vi "Fixed Point.vi"() -> (3 "Unit Test Framework Results":T1)   [LabVIEW 2015]
doc: "Use this template to create a user-defined test VI. Define your test requirements and wire the results to the <b>Result (Test)</b> control. Do not modify the <b>Unit Test Framework Results</b> indicator."
uses:
  <vilib>/utf/common/utf_test_result_troll.ctl
  <vilib>/utf/common/utf_test_result.ctl
  <vilib>/utf/common/utf_test_result_failure.ctl
  <vilib>/utf/common/utf_test_comparison_operators.ctl
  <vilib>/utf/common/utf_vi_tag.ctl
  <userlib>/LV Test Utils v1/LV Test Utils.lvlib
  <vilib>/utf/NI_UnitTestFramework.lvlib
panel:
  out "string":string
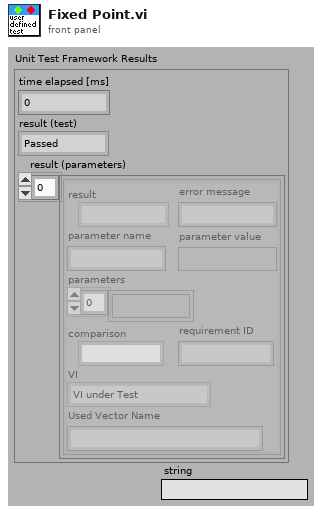
[diagram p1: front panel]
types:
  T1 = typedef "NI_UnitTestFramework.lvlib/utf_test_result_troll.ctl" = cluster{"time elapsed [ms]":u32, "result (test)":T2, "result (parameters)":T3[]}
  T2 = typedef "NI_UnitTestFramework.lvlib/utf_test_result.ctl" = enum16{"Passed", "Failed", "Error", "Skipped", "Not Processed"}
  T3 = typedef "NI_UnitTestFramework.lvlib/utf_test_result_failure.ctl" = cluster{"result":T2, "error message":string, "parameter name":string, "parameter value":variant, "parameters":variant[], "comparison":T4, "requirement ID":string, "VI":T5, "Used Vector Name":string}
  T4 = typedef "NI_UnitTestFramework.lvlib/utf_test_comparison_operators.ctl" = enum16{"=", "!=", ">", ">=", "<", "<=", "range", "symmetric tolerance", "asymmetric tolerance", "string contains", "string not contain", "array size", "string length", "array range", "by element", "array range (limit array)", "user-defined", "array contains", "array not contain", "vector length", "= (elm)", "!= (elm)", "= (case insensitive)", "!= (case insensitive)"}
  T5 = typedef "NI_UnitTestFramework.lvlib/utf_vi_tag.ctl" = enum16{"Setup VI", "VI under Test", "Teardown VI"}
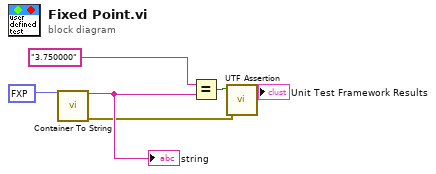
[diagram p0: block diagram]
diagram:
  n1 = call "Container To String.vi"("variant"=fxp<+,4,2> 3.75) -> ("string"=w5:string, "error out"=w2:errorcluster)  [unwired: 12 in, 1 out]
  "string" <- w5
  n2 = Equal?(x="3.750000" ("string"), y=w5) -> (x = y?=w3:bool)
  n3 = call <userlib>:"UTF Assertion.vi"("error in"=w2, "assertion"=w3) -> ("Unit Test Framework - Result"=→"Unit Test Framework Results":T1)  [unwired: 3 in]
